vi "Device Level, Process Pulses.vi"(6 "error in":errorcluster, 7 "Average Size":dbl=15.0, 8 "Resistance (ohms)":dbl=500.0 format="%.1f", 9 "waveform":waveform(dbl)={"t0"=timestamp(3473168073.631 s since 1904-01-01), "dt"=1e-08, "Y"=[]}) -> (0 "error out":errorcluster, 1 "Input Parameters":T1[](array[typedef]) {"Value" format="%#.3f"}, 2 "Results":T1[](array[typedef]) {"Value" format="%#.3f"}, 3 "waveform out":waveform(dbl)={"t0"=timestamp(3472747248.0780005 s since 1904-01-01), "dt"=nan, "Y"=[]})   [LabVIEW 2010]
doc: "This function processes a multi-pulse waveform to determine the Stimulus Amplitude, Stimulus Pulse Width, Recovery Amplitude, Recovery Pulse Width, Interphase Delay, and Pulse Repetition Frequency.\n\nResults are stored as Waveform attributes and to an array of clusters."
uses:
  Generic/Waveform Attribute/Waveform Attribute Cluster.ctl
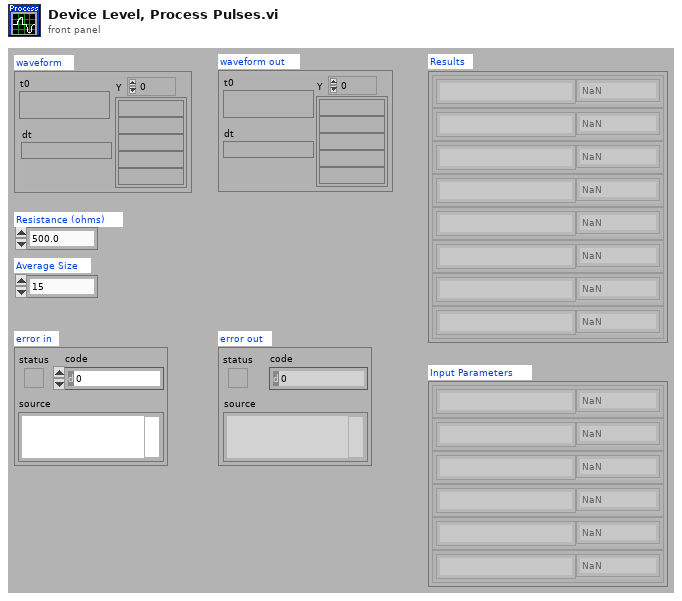
[diagram p1: front panel]
types:
  T1 = typedef "Waveform Attribute Cluster.ctl" = cluster{"Label":string, "Value":dbl}
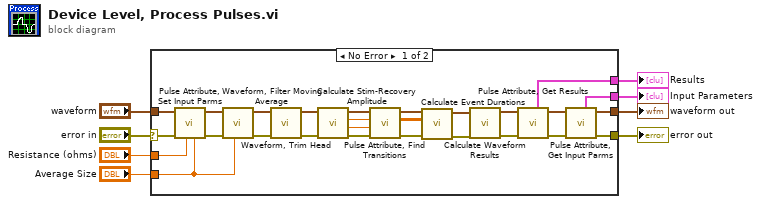
[diagram p0: block diagram]
diagram:
  n1 = case shown="No Error" "error in" {
    selector: "error in" -> [w35 w36]
    tunnel: [w30 w36] -> w8
    tunnel: "Average Size" -> [w32 _]
    tunnel: "waveform" -> [w28 _]
    tunnel: "Resistance (ohms)" -> [w31 _]
    tunnel: [w26 _] -> w3
    tunnel: [w27 _] -> w2
    tunnel: [w22 _] -> w1
    frame No Error {
      n2 = call "Pulse Attribute, Set Input Parms.vi"("Average Size"=w32, "Resistance (ohms)"=w31, "error in"=w35, "waveform"=w28) -> ("error out"=w34:errorcluster, "waveform out"=w33:waveform(dbl))  [unwired: 4 in]
      n3 = call "Waveform, Filter Moving Average.vi"("Average Size"=w32, "error in"=w34, "waveform"=w33) -> ("error out"=w21:errorcluster, "waveform out"=w19:waveform(dbl))  [unwired: 5 in]
      n4 = call "Waveform, Trim Head.vi"("error in"=w21, "waveform"=w19) -> ("error out"=w20:errorcluster, "waveform out"=w18:waveform(dbl))  [unwired: 6 in, 1 out]
      n5 = call "Calculate Stim-Recovery Amplitude.vi"("error in"=w20, "waveform"=w18) -> ("error out"=w17:errorcluster, "Recvy Amp (V)"=w14:dbl, "Stim Amp (V)"=w15:dbl, "waveform out"=w16:waveform(dbl))  [unwired: 6 in]
      n6 = call "Pulse Attribute, Find Transitions.vi"("error in"=w17, "Recvy Amp (V)"=w14, "Stim Amp (V)"=w15, "waveform"=w16) -> ("error out"=w13:errorcluster, "transitions"=w9:dbl[][], "waveform dup"=w12:waveform(dbl))  [unwired: 5 in]
      n7 = call "Calculate Event Durations.vi"("error in"=w13, "transitions"=w9, "waveform"=w12) -> ("error out"=w11:errorcluster, "waveform out"=w10:waveform(dbl))  [unwired: 7 in]
      n8 = call "Calculate Waveform Results.vi"("error in"=w11, "waveform in"=w10) -> ("error out"=w24:errorcluster, "waveform out"=w23:waveform(dbl))  [unwired: 8 in]
      n9 = call "Pulse Attribute, Get Results.vi"("error in"=w24, "waveform"=w23) -> ("error out"=w25:errorcluster, "waveform dup"=w29:waveform(dbl), "Results"=w27:T1[])  [unwired: 5 in]
      n10 = call "Pulse Attribute, Get Input Parms.vi"("error in"=w25, "waveform"=w29) -> ("error out"=w30:errorcluster, "waveform dup"=w22:waveform(dbl), "input parameters"=w26:T1[])  [unwired: 5 in]
    }
    frame Error {
    }
  }
  "error out" <- w8
  "Results" <- w2
  "waveform out" <- w1
  "Input Parameters" <- w3
